vi "Shift Register Delay.vi"(1 "input":dbl format="%.2f", 2 "n delay (0)":i32) -> (0 "output":dbl format="%.2f")   [LabVIEW 2023]
doc: "An uninitialized shift register is used as a delay element. N Delay chooses the mutiplier on the delay, from 0 (no delay) to 10 (maximum delay). After the input changes, on the Nth call of this VI that change will appear at the output. The VI is reentrant, so you can call it from several locations without interference."
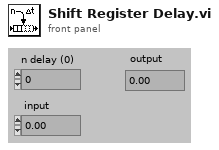
[diagram p1: front panel]
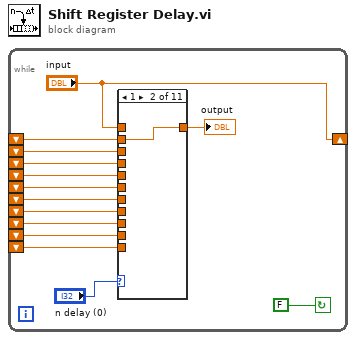
[diagram p0: block diagram]
diagram:
  n1 = while {
    shift-left: _ -> [w11]
    shift-left: _ -> [w10]
    shift-left: _ -> [w9]
    shift-left: _ -> [w8]
    shift-left: _ -> [w7]
    shift-left: _ -> [w6]
    shift-left: _ -> [w5]
    shift-left: _ -> [w4]
    shift-left: _ -> [w3]
    shift-left: _ -> [w12]
    shift-right: ["input"] -> _
    stop <- FALSE continue-if-true
    n2 = case shown="1" "n delay (0)" {
      tunnel: w3 -> [_ _ _ _ _ _ _ _ _ _ w25]
      tunnel: w4 -> [_ _ _ _ _ _ _ _ _ w24 _]
      tunnel: w5 -> [_ _ _ _ _ _ _ _ w23 _ _]
      tunnel: w6 -> [_ _ _ _ _ _ _ w22 _ _ _]
      tunnel: w7 -> [_ _ _ _ _ _ w21 _ _ _ _]
      tunnel: w8 -> [_ _ _ _ _ w20 _ _ _ _ _]
      tunnel: w9 -> [_ _ _ _ w19 _ _ _ _ _ _]
      tunnel: w10 -> [_ _ _ w18 _ _ _ _ _ _ _]
      tunnel: w11 -> [_ _ w17 _ _ _ _ _ _ _ _]
      tunnel: w12 -> [_ w16 _ _ _ _ _ _ _ _ _]
      tunnel: "input" -> [w15 _ _ _ _ _ _ _ _ _ _]
      tunnel: [w15 w16 w17 w18 w19 w20 w21 w22 w23 w24 w25] -> w2
      frame ..0 {
      }
      frame 1 {
      }
      frame 2 {
      }
      frame 3 {
      }
      frame 4 {
      }
      frame 5 {
      }
      frame 6 {
      }
      frame 7 {
      }
      frame 8 {
      }
      frame 9 {
      }
      frame 10.. {
      }
    }
    "output" <- w2
  }
